vi "algo.vi"(8 "debug":bool, 11 "reset":bool) -> (1 "Ready.for.OrderBook.Command.Input":bool, 2 "Ready.for.Configuration.Input":bool)   [LabVIEW 2022 SP3]
uses:
  types/algo.states.ctl
  types/algo.mode.ctl
  types/algo.scratch.ctl
  algo.data.ctl
  common/orderbook.command.type.ctl
  common/orderbook.command.ctl
  types/algo.stats.ctl
  types/algo.cmd.debug.ctl
  types/algo.cmd.state.ctl
  types/algo.cmd.mem.orders.ctl
  types/algo.cmd.mem.watchlist.ctl
  types/algo.val.state.ctl
  types/algo.val.debug.ctl
  types/algo.time.ctl
  types/algo.algo.ctl
  types/algo.val.watchlist.ctl
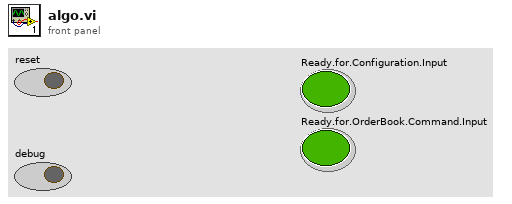
[diagram p1: front panel]
types:
  T1 = typedef "algo.states.ctl" = enum16{"Noop", "Reset", "Configuration", "Debug", "Get.State", "Wait.for.Command", "Process.Add", "Process.Edit", "Process.Remove"}
  T2 = typedef "algo.data.ctl" = cluster{"next.state":T1, "saved.state":T1, "scratch":T3, "mode":T4, "memory.watchlist":T5, "memory.orders":T7, "state":T8, "debug":T10, "stats":T12, "orderbook.command":T13, "algo":T15, "time":T16}
  T3 = typedef "algo.scratch.ctl" = cluster{"i":u64, "n":u64, "start.addr":u16, "first.call?":bool}
  T4 = typedef "algo.mode.ctl" = enum16{"GetLoc", "Start", "Search", "Shift"}
  T5 = typedef "algo.cmd.mem.watchlist.ctl" = cluster{"read.addr":u16, "read.request":bool, "read.ready":bool, "write.addr":u16, "write.request":bool, "val.watchlist.read":T6, "val.watchlist.write":T6}
  T6 = typedef "algo.val.watchlist.ctl" = cluster{"symbol":u64, "buy.size":u16, "buy.start.addr":u16, "sell.start.addr":u16, "sell.size":u16, "min.ask":u32, "max.bid":u32}
  T7 = typedef "algo.cmd.mem.orders.ctl" = cluster{"read.addr":u16, "read.data":cluster{"value":u64}, "read.request":bool, "read.ready":bool, "write.addr":u16, "write.request":bool, "write.data":cluster{"value":u64}}
  T8 = typedef "algo.cmd.state.ctl" = cluster{"write.to.state":bool, "val.state":T9}
  T9 = typedef "algo.val.state.ctl" = u64[]
  T10 = typedef "algo.cmd.debug.ctl" = cluster{"write.to.debug":bool, "val.debug":T11}
  T11 = typedef "algo.val.debug.ctl" = u64[]
  T12 = typedef "algo.stats.ctl" = cluster{"min.ask":u32, "max.bid":u32, "price":u32, "quantity":u32, "execution":bool}
  T13 = typedef "orderbook.command.ctl" = cluster{"type":T14, "side":u8, "orderId ":u64, "quantity":u32, "symbol":u64, "price":u64, "executed.qty":u32, "canceled.qty":u32, "remaining.qty":u32, "seconds":u64, "nanoseconds":u64}
  T14 = typedef "orderbook.command.type.ctl" = enum8{"Time", "AddOrder", "OrderExecuted", "OrderExecutedAtPrice", "ReduceSize", "ModifyOrder", "DeleteOrder", "Get.State", "Get.All.Orders", "Get.Top"}
  T15 = typedef "algo.algo.ctl" = cluster{"min.ask":u32, "max.bid":u32}
  T16 = typedef "algo.time.ctl" = cluster{"last":u32, "since":u32}
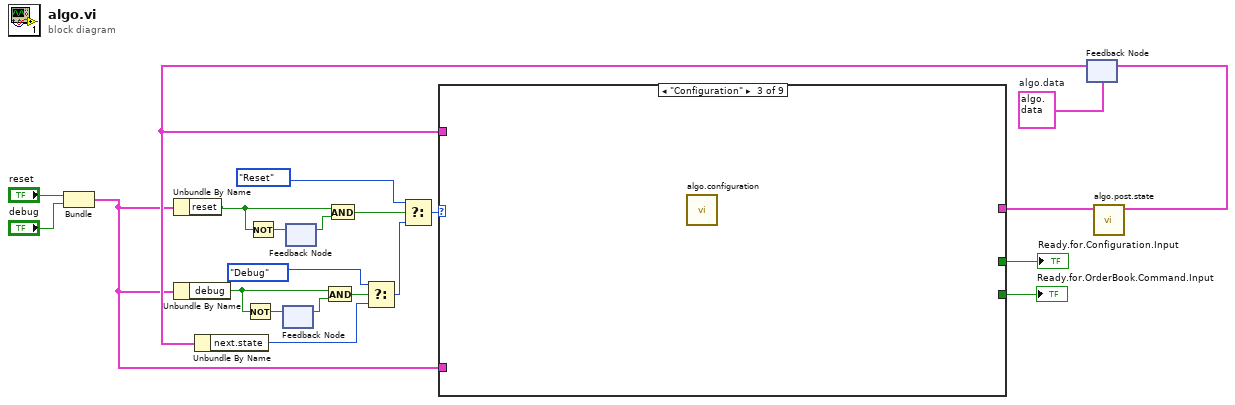
[diagram p0: block diagram]
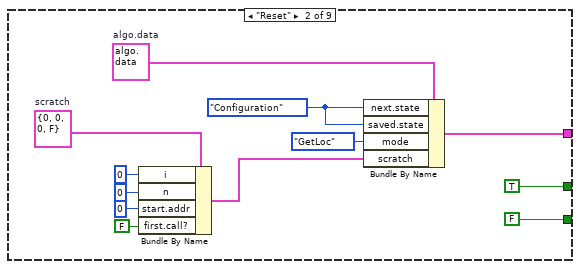
[diagram p3: hidden frame]
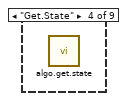
[diagram p4: hidden frame]
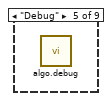
[diagram p5: hidden frame]
diagram:
  w6 = T2 {"next.state"=enum."Wait.for.Command", "saved.state"=enum."Wait.for.Command", "scratch"={"i"=0, "n"=0, "start.addr"=0, "first.call?"=FALSE}, "mode"=enum."GetLoc", "memory.watchlist"={"read.addr"=0, "read.request"=FALSE, "read.ready"=FALSE, "write.addr"=0, "write.request"=FALSE, "val.watchlist.read"={"symbol"=0, "buy.size"=0, "buy.start.addr"=0, "sell.start.addr"=0, "sell.size"=0, "min.ask"=0, "max.bid"=0}, "val.watchlist.write"={"symbol"=0, "buy.size"=0, "buy.start.addr"=0, "sell.start.addr"=0, "sell.size"=0, "min.ask"=0, "max.bid"=0}}, "memory.orders"={"read.addr"=0, "read.data"={"value"=0}, "read.request"=FALSE, "read.ready"=FALSE, "write.addr"=0, "write.request"=FALSE, "write.data"={"value"=0}}, "state"={"write.to.state"=FALSE, "val.state"=[0, 0]}, "debug"={"write.to.debug"=FALSE, "val.debug"=[0, 0]}, "stats"={"min.ask"=0, "max.bid"=0, "price"=0, "quantity"=0, "execution"=FALSE}, "orderbook.command"={"type"=enum."AddOrder", "side"=0, "orderId "=0, "quantity"=0, "symbol"=0, "price"=0, "executed.qty"=0, "canceled.qty"=0, "remaining.qty"=0, "seconds"=0, "nanoseconds"=0}, "algo"={"min.ask"=0, "max.bid"=0}, "time"={"last"=0, "since"=0}}  # algo.data
  n1 = Bundle("reset"="reset", "debug"="debug") -> (w7:cluster{"reset":bool, "debug":bool})  [unwired: 1 in]
  n2 = Unbundle By Name(w7) -> ("reset"=w19:bool)
  n3 = Unbundle By Name(w7) -> ("debug"=w16:bool)
  n4 = Not(x=w16) -> (.not. x?=w18:bool)
  n5 = Not(x=w19) -> (.not. x?=w21:bool)
  n6 = feedback #1() -> (w17:bool)  [unwired: 1 in]
  n7 = feedback-in #1(w18) -> ()
  n8 = feedback #2() -> (w20:bool)  [unwired: 1 in]
  n9 = feedback-in #2(w21) -> ()
  n10 = And(x=w16, y=w17) -> (x .and. y?=w14:bool)
  n11 = And(x=w19, y=w20) -> (x .and. y?=w15:bool)
  n12 = feedback #3(w6) -> (w10:T2)
  n13 = Unbundle By Name(w10) -> ("next.state"=w12:T1)
  n14 = Select(t=algo.states."Debug" ("algo.states"), s=w14, f=w12) -> (s? t:f=w13:T1)
  n15 = Select(t=algo.states."Reset" ("algo.states"), s=w15, f=w13) -> (s? t:f=w11:T1)
  n16 = case shown="\"Configuration\"" w11 {
    tunnel: [w23 w35 _ _ _ _ _ _ _] -> w4
    tunnel: w10 -> [w23 _ _ _ _ _ _ _ _]
    tunnel: [_ TRUE _ _ _ _ _ _ _] -> w9
    tunnel: [_ FALSE _ _ _ _ _ _ _] -> w8
    tunnel: w7 -> [_ _ _ _ _ _ _ _ _]
    frame "Noop", Default {
    }
    frame "Reset" {
      w27 = algo.states."Configuration" ("state")
      w31 = T3 {"i"=0, "n"=0, "start.addr"=0, "first.call?"=FALSE}  # scratch
      w32 = T2 {"next.state"=enum."Wait.for.Command", "saved.state"=enum."Wait.for.Command", "scratch"={"i"=0, "n"=0, "start.addr"=0, "first.call?"=FALSE}, "mode"=enum."GetLoc", "memory.watchlist"={"read.addr"=0, "read.request"=FALSE, "read.ready"=FALSE, "write.addr"=0, "write.request"=FALSE, "val.watchlist.read"={"symbol"=0, "buy.size"=0, "buy.start.addr"=0, "sell.start.addr"=0, "sell.size"=0, "min.ask"=0, "max.bid"=0}, "val.watchlist.write"={"symbol"=0, "buy.size"=0, "buy.start.addr"=0, "sell.start.addr"=0, "sell.size"=0, "min.ask"=0, "max.bid"=0}}, "memory.orders"={"read.addr"=0, "read.data"={"value"=0}, "read.request"=FALSE, "read.ready"=FALSE, "write.addr"=0, "write.request"=FALSE, "write.data"={"value"=0}}, "state"={"write.to.state"=FALSE, "val.state"=[0, 0]}, "debug"={"write.to.debug"=FALSE, "val.debug"=[0, 0]}, "stats"={"min.ask"=0, "max.bid"=0, "price"=0, "quantity"=0, "execution"=FALSE}, "orderbook.command"={"type"=enum."AddOrder", "side"=0, "orderId "=0, "quantity"=0, "symbol"=0, "price"=0, "executed.qty"=0, "canceled.qty"=0, "remaining.qty"=0, "seconds"=0, "nanoseconds"=0}, "algo"={"min.ask"=0, "max.bid"=0}, "time"={"last"=0, "since"=0}}  # algo.data
      n17 = Bundle By Name(cluster=w31, "i"=u64 0 ("I"), "n"=u64 0 ("N"), "start.addr"=u16 0, "first.call?"=FALSE ("FirstCall?")) -> (w25:T3)
      n18 = Bundle By Name(cluster=w32, "next.state"=w27, "saved.state"=w27, "mode"=algo.mode."GetLoc", "scratch"=w25) -> (w35:T2)
    }
    frame "Configuration" {
      n19 = call "algo.configuration.vi"() -> ()  [unwired: 12 in]
    }
    frame "Get.State" {
      n20 = call "algo.get.state.vi"() -> ()  [unwired: 12 in]
    }
    frame "Debug" {
      n21 = call "algo.debug.vi"() -> ()  [unwired: 12 in]
    }
    frame "Wait.for.Command" {
    }
    frame "Process.Add" {
    }
    frame "Process.Edit" {
    }
    frame "Process.Remove" {
    }
  }
  "Ready.for.OrderBook.Command.Input" <- w8
  "Ready.for.Configuration.Input" <- w9
  n22 = call "algo.post.state.vi"("algo.data.in"=w4) -> ("algo.data.out"=w5:T2)  [unwired: 10 in]
  n23 = feedback-in #3(w5) -> ()
